vi "InitDev.vi"(1 "SAVE?":bool, 2 "IP地址":string="192.168.1.16", 3 "SavePath":path) -> (0 "输出簇":T1)   [LabVIEW 2012]
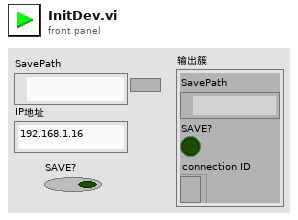
[diagram p1: front panel]
types:
  T1 = cluster{"SavePath":path, "SAVE?":bool, "connection ID":refnum<k5>}
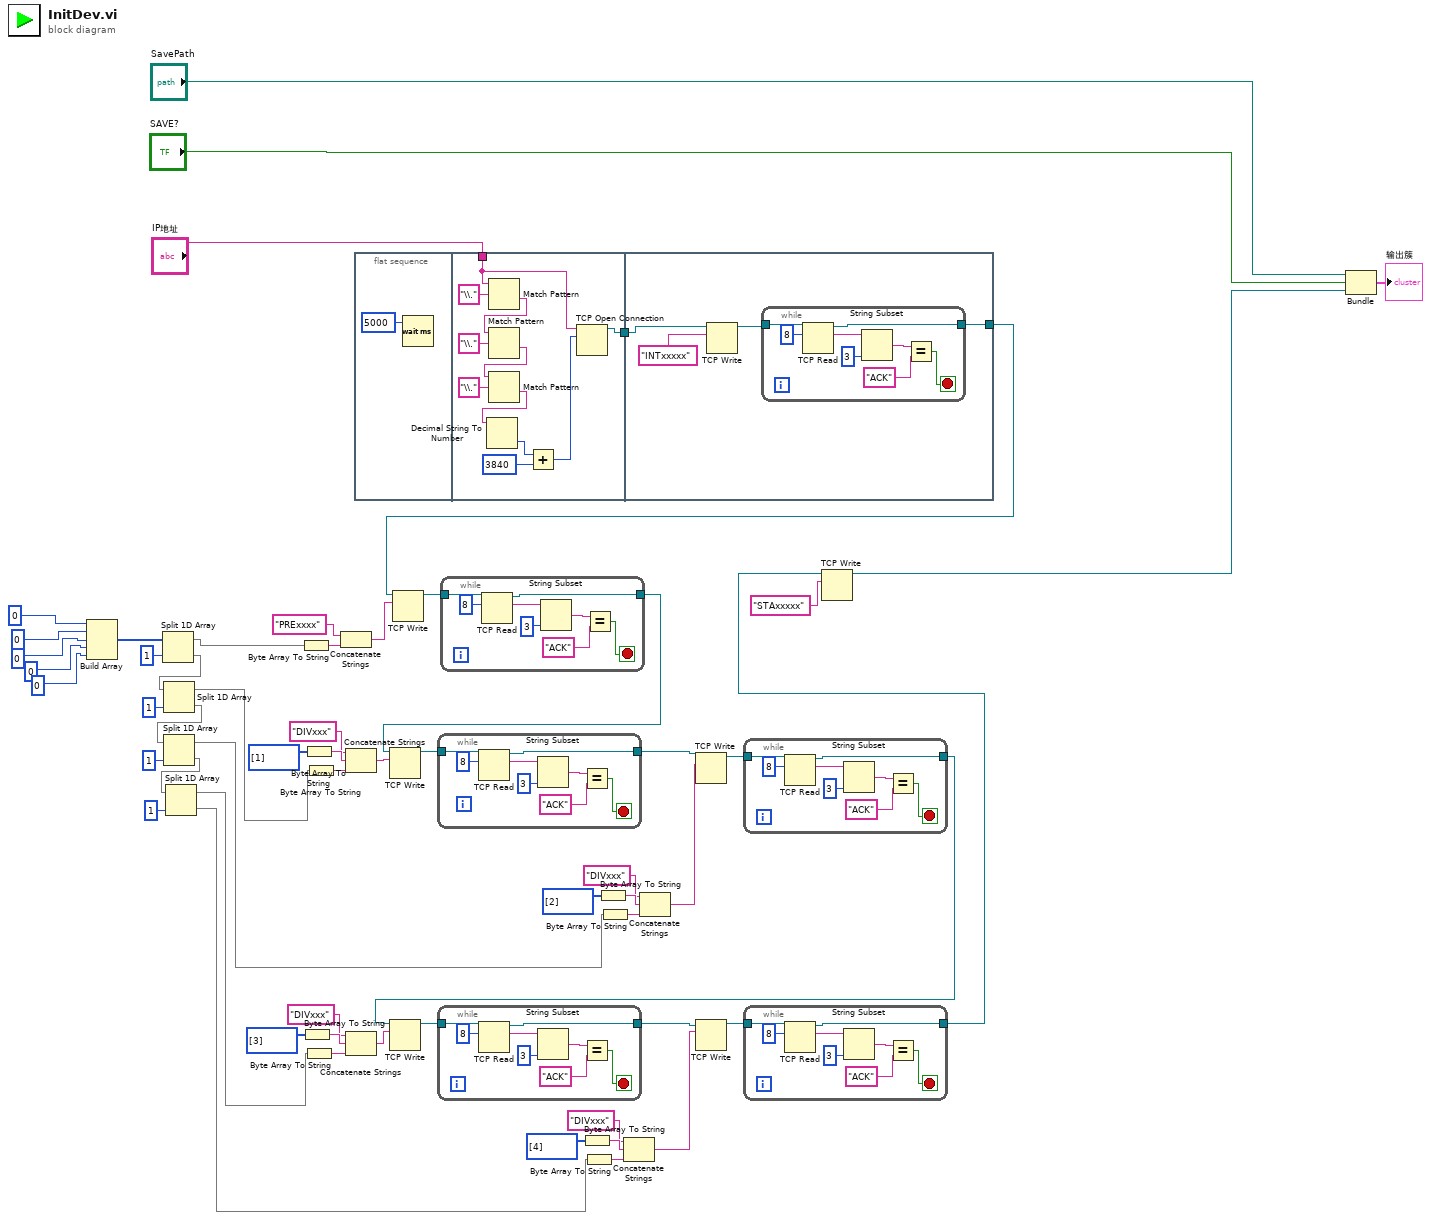
[diagram p0: block diagram]
diagram:
  n1 = Build Array(u8 0 ("元素"), u8 0 ("元素"), u8 0 ("元素"), u8 0 ("元素"), u8 0 ("元素")) -> (w58:u8[])
  n2 = Split 1D Array(array=w58, index=1 ("索引")) -> (first subarray=w39:u8[], second subarray=w35:u8[])
  n3 = Split 1D Array(array=w35, index=1 ("索引")) -> (first subarray=w15:u8[], second subarray=w34:u8[])
  n4 = Split 1D Array(array=w34, index=1 ("索引")) -> (first subarray=w14:u8[], second subarray=w33:u8[])
  n5 = Split 1D Array(array=w33, index=1 ("索引")) -> (first subarray=w13:u8[], second subarray=w12:u8[])
  n6 = Byte Array To String(unsigned byte array=w39) -> (string=w43:string)
  n7 = Byte Array To String(unsigned byte array=u8[] [3] ("无符号字节数组")) -> (string=w21:string)
  n8 = Byte Array To String(unsigned byte array=u8[] [1] ("无符号字节数组")) -> (string=w29:string)
  n9 = Byte Array To String(unsigned byte array=w13) -> (string=w23:string)
  n10 = Byte Array To String(unsigned byte array=w15) -> (string=w32:string)
  n11 = Concatenate Strings("PRExxxx" ("数据输入"), w43) -> (w41:string)
  n12 = Concatenate Strings("DIVxxx" ("数据输入"), w29, w32) -> (w31:string)
  n13 = Concatenate Strings("DIVxxx" ("数据输入"), w21, w23) -> (w7:string)
  n14 = flat-sequence {
    tunnel: [w71] -> w59
    tunnel: "IP地址" -> [w62]
    tunnel: w59 -> [w74]
    tunnel: [w72] -> w6
    frame #0 {
      n15 = Wait (ms)(milliseconds to wait=u32 5000 ("毫秒倍数")) -> ()  [unwired: 1 out]
    }
    frame #1 {
      n16 = Match Pattern(string=w62, regular expression="\\." ("正则表达式")) -> (after substring=w66:string)  [unwired: 1 in, 3 out]
      n17 = Match Pattern(string=w66, regular expression="\\." ("正则表达式")) -> (after substring=w67:string)  [unwired: 1 in, 3 out]
      n18 = Match Pattern(string=w67, regular expression="\\." ("正则表达式")) -> (after substring=w68:string)  [unwired: 1 in, 3 out]
      n19 = Decimal String To Number(string=w68) -> (number=w69:i32)  [unwired: 2 in, 1 out]
      n20 = Add(x=w69, y=3840) -> (x+y=w61:i32)
      n21 = TCP Open Connection(address=w62, remote port or service name=w61) -> (connection ID=w71:refnum<k5>)  [unwired: 3 in, 1 out]
    }
    frame #2 {
      n22 = TCP Write(connection ID=w74, data in="INTxxxxx" ("数据输入")) -> (connection ID out=w73:refnum<k5>)  [unwired: 2 in, 2 out]
      n23 = while {
        tunnel: w73 -> [w83]
        tunnel: [w77] -> w72
        stop <- w78 stop-if-true
        n24 = TCP Read(connection ID=w83, bytes to read=8 ("读取的字节")) -> (connection ID out=w77:refnum<k5>, data out=w81:string)  [unwired: 3 in, 1 out]
        n25 = String Subset(string=w81, length (rest)=3 ("偏移量(0)")) -> (substring=w80:string)  [unwired: 1 in]
        n26 = Equal?(x=w80, y="ACK") -> (x = y?=w78:bool)
      }
    }
  }
  n27 = TCP Write(connection ID=w6, data in=w41) -> (connection ID out=w52:refnum<k5>)  [unwired: 2 in, 2 out]
  n28 = while {
    tunnel: w52 -> [w91]
    tunnel: [w85] -> w47
    stop <- w86 stop-if-true
    n29 = TCP Read(connection ID=w91, bytes to read=8 ("读取的字节")) -> (connection ID out=w85:refnum<k5>, data out=w89:string)  [unwired: 3 in, 1 out]
    n30 = String Subset(string=w89, length (rest)=3 ("偏移量(0)")) -> (substring=w88:string)  [unwired: 1 in]
    n31 = Equal?(x=w88, y="ACK") -> (x = y?=w86:bool)
  }
  n32 = TCP Write(connection ID=w47, data in=w31) -> (connection ID out=w51:refnum<k5>)  [unwired: 2 in, 2 out]
  n33 = while {
    tunnel: w51 -> [w99]
    tunnel: [w93] -> w46
    stop <- w94 stop-if-true
    n34 = TCP Read(connection ID=w99, bytes to read=8 ("读取的字节")) -> (connection ID out=w93:refnum<k5>, data out=w97:string)  [unwired: 3 in, 1 out]
    n35 = String Subset(string=w97, length (rest)=3 ("偏移量(0)")) -> (substring=w96:string)  [unwired: 1 in]
    n36 = Equal?(x=w96, y="ACK") -> (x = y?=w94:bool)
  }
  n37 = Byte Array To String(unsigned byte array=u8[] [4] ("无符号字节数组")) -> (string=w17:string)
  n38 = Byte Array To String(unsigned byte array=w12) -> (string=w19:string)
  n39 = Byte Array To String(unsigned byte array=u8[] [2] ("无符号字节数组")) -> (string=w25:string)
  n40 = Byte Array To String(unsigned byte array=w14) -> (string=w27:string)
  n41 = Concatenate Strings("DIVxxx" ("数据输入"), w17, w19) -> (w10:string)
  n42 = Concatenate Strings("DIVxxx" ("数据输入"), w25, w27) -> (w11:string)
  n43 = TCP Write(connection ID=w46, data in=w11) -> (connection ID out=w50:refnum<k5>)  [unwired: 2 in, 2 out]
  n44 = while {
    tunnel: w50 -> [w107]
    tunnel: [w101] -> w45
    stop <- w102 stop-if-true
    n45 = TCP Read(connection ID=w107, bytes to read=8 ("读取的字节")) -> (connection ID out=w101:refnum<k5>, data out=w105:string)  [unwired: 3 in, 1 out]
    n46 = String Subset(string=w105, length (rest)=3 ("偏移量(0)")) -> (substring=w104:string)  [unwired: 1 in]
    n47 = Equal?(x=w104, y="ACK") -> (x = y?=w102:bool)
  }
  n48 = TCP Write(connection ID=w45, data in=w7) -> (connection ID out=w49:refnum<k5>)  [unwired: 2 in, 2 out]
  n49 = while {
    tunnel: w49 -> [w115]
    tunnel: [w109] -> w44
    stop <- w110 stop-if-true
    n50 = TCP Read(connection ID=w115, bytes to read=8 ("读取的字节")) -> (connection ID out=w109:refnum<k5>, data out=w113:string)  [unwired: 3 in, 1 out]
    n51 = String Subset(string=w113, length (rest)=3 ("偏移量(0)")) -> (substring=w112:string)  [unwired: 1 in]
    n52 = Equal?(x=w112, y="ACK") -> (x = y?=w110:bool)
  }
  n53 = TCP Write(connection ID=w44, data in=w10) -> (connection ID out=w48:refnum<k5>)  [unwired: 2 in, 2 out]
  n54 = while {
    tunnel: w48 -> [w123]
    tunnel: [w117] -> w9
    stop <- w118 stop-if-true
    n55 = TCP Read(connection ID=w123, bytes to read=8 ("读取的字节")) -> (connection ID out=w117:refnum<k5>, data out=w121:string)  [unwired: 3 in, 1 out]
    n56 = String Subset(string=w121, length (rest)=3 ("偏移量(0)")) -> (substring=w120:string)  [unwired: 1 in]
    n57 = Equal?(x=w120, y="ACK") -> (x = y?=w118:bool)
  }
  n58 = TCP Write(connection ID=w9, data in="STAxxxxx" ("数据输入")) -> (connection ID out=w4:refnum<k5>)  [unwired: 2 in, 2 out]
  n59 = Bundle("SavePath"="SavePath", "SAVE?"="SAVE?", "connection ID"=w4) -> (→"输出簇":T1)  [unwired: 1 in]
